vi "Dynamic Generation of Formula for Vtip.vi"(11 "Voltage (V)":T1={"Schedule"=enum."Constant", "Value"=10.0, "Start Value"=0.0, "End Value"=0.0, "Min Value"=0.0, "Max Value"=0.0, "Duty Cycle (%)"=0.0, "Signal Type"=enum."Square Wave", "Cycle Number"=0.0, "Phase (degrees)"=0.0, "formula"="1*(step(170-t)*cos(0.62831853071*t)+step(t-170)*cos(0.62831853071*(t-170))*(-1))", "formula length (nm)"=340.0, "formula resolution (nm)"=0.001}) -> (3 "Voltage (V) 2":T1={"Schedule"=enum."Constant", "Value"=10.0, "Start Value"=0.0, "End Value"=0.0, "Min Value"=0.0, "Max Value"=0.0, "Duty Cycle (%)"=0.0, "Signal Type"=enum."Square Wave", "Cycle Number"=0.0, "Phase (degrees)"=0.0, "formula"="1*(step(170-t)*cos(0.62831853071*t)+step(t-170)*cos(0.62831853071*(t-170))*(-1))", "formula length (nm)"=340.0, "formula resolution (nm)"=0.001})   [LabVIEW 2016]
uses:
  typedefs/Voltage - cluster.ctl
  typedefs/Schedule - enum.ctl
  typedefs/Signal Type - enum.ctl
  <vilib>/gmath/NI_Gmath.lvlib
panel:
  out "error":i32
  in  "formula":string="1*(step(170-t)*cos(0.62831853071*t)+step(t-170)*cos(0.62831853071*(t-170))*(-1))"
  out "XY Graph":cluster{"X Values":dbl[], "Y Values":dbl[]}(graph)
  in  "Resolution (nm)":dbl=0.001
  in  "Length (nm)":dbl=340.0
  in  "OK":bool
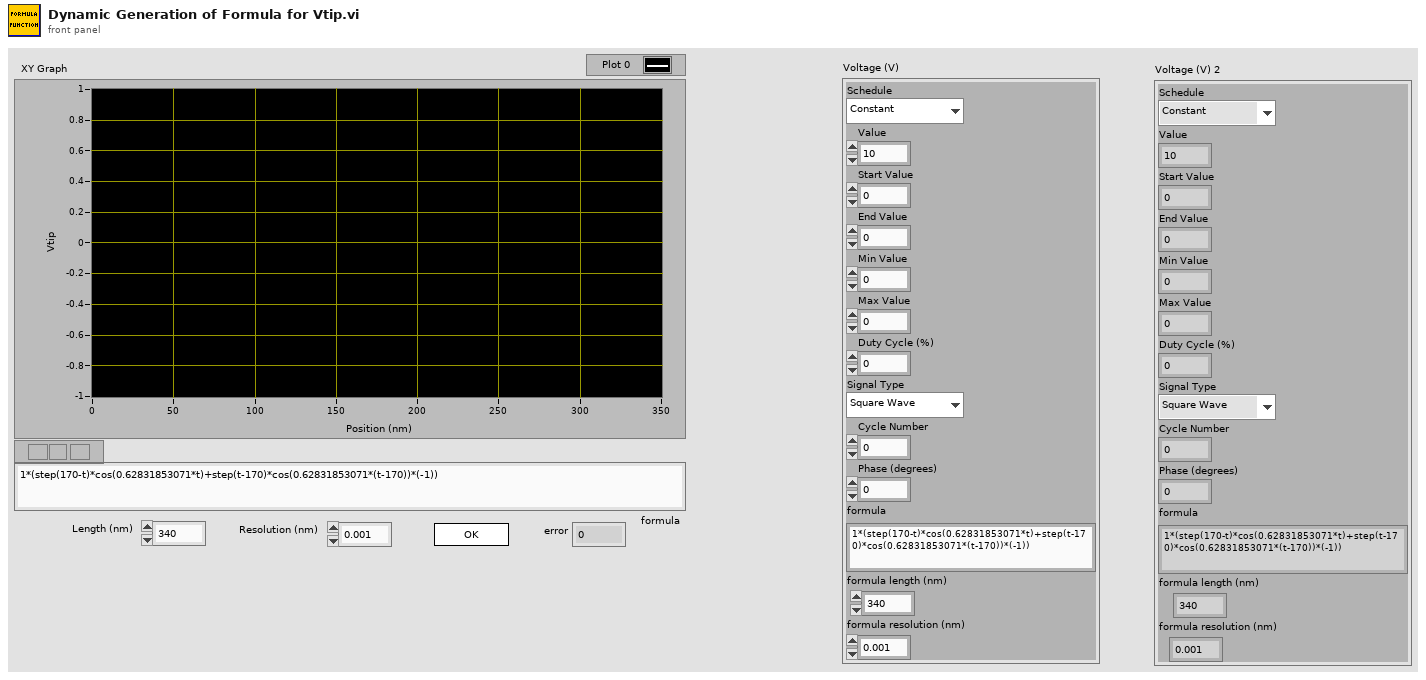
[diagram p1: front panel]
types:
  T1 = typedef "Voltage - cluster.ctl" = cluster{"Schedule":T2, "Value":dbl, "Start Value":dbl, "End Value":dbl, "Min Value":dbl, "Max Value":dbl, "Duty Cycle (%)":dbl, "Signal Type":T3, "Cycle Number":dbl, "Phase (degrees)":dbl, "formula":string, "formula length (nm)":dbl, "formula resolution (nm)":dbl}
  T2 = typedef "Schedule - enum.ctl" = enum16{"Constant", "Ramp", "Fn. Generator", "Formula"}
  T3 = typedef "Signal Type - enum.ctl" = enum16{"Sine Wave", "Triangle Wave", "Square Wave", "Sawtooth Wave"}
  T4 = enum32{"invalid app kind", "Development System", "Run Time System", "Student Edition", "Embedded LabVIEW", "Evaluation", "Custom"}
  T5 = enum32{"Invalid", "Standard", "Closed", "Hidden", "Minimized", "Maximized"}
  T6 = cluster{"Core":cluster{"Current VI Reference":refnum<vi>, "Close Panel on Exit?":bool}, "Your Boolean data":bool, "Your string data":string, "#s":u32, "Voltage (V)":T1}
  T7 = cluster{"Current VI Reference":refnum<vi>, "Close Panel on Exit?":bool}
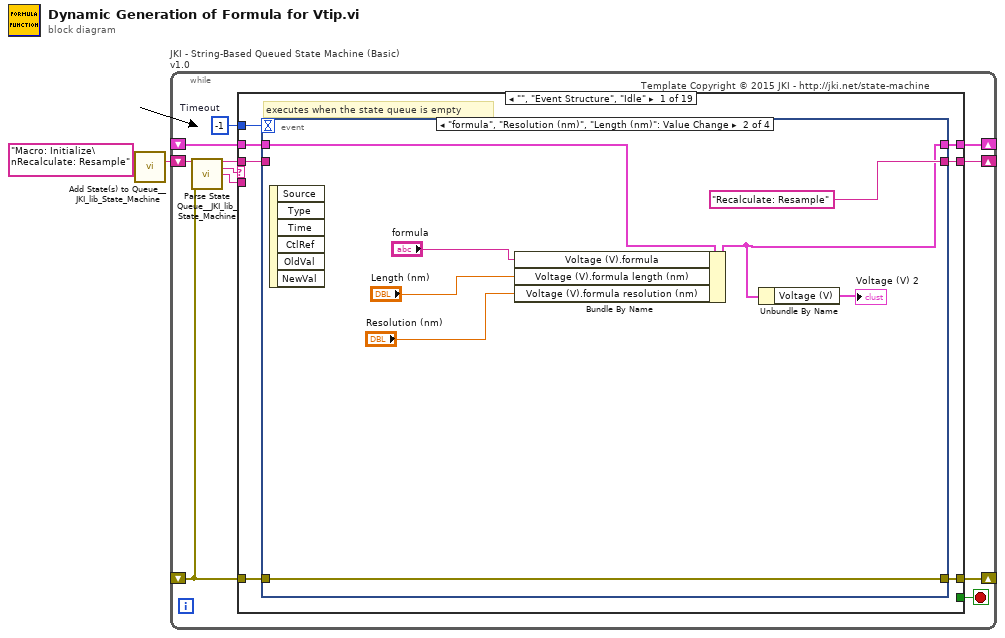
[diagram p0: block diagram]
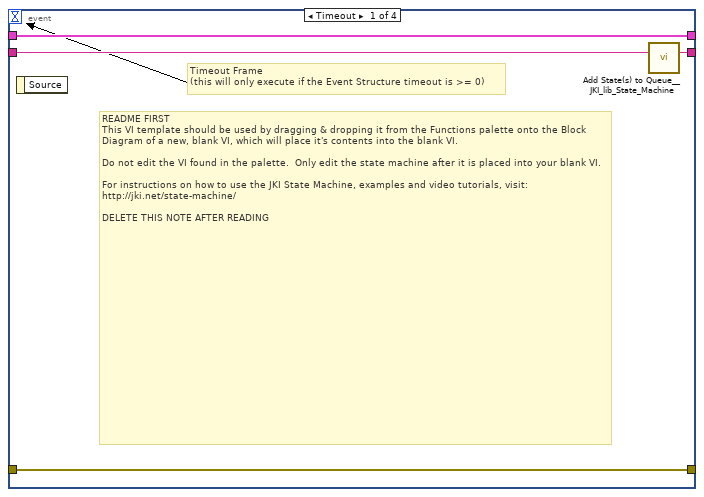
[diagram p2: hidden frame]
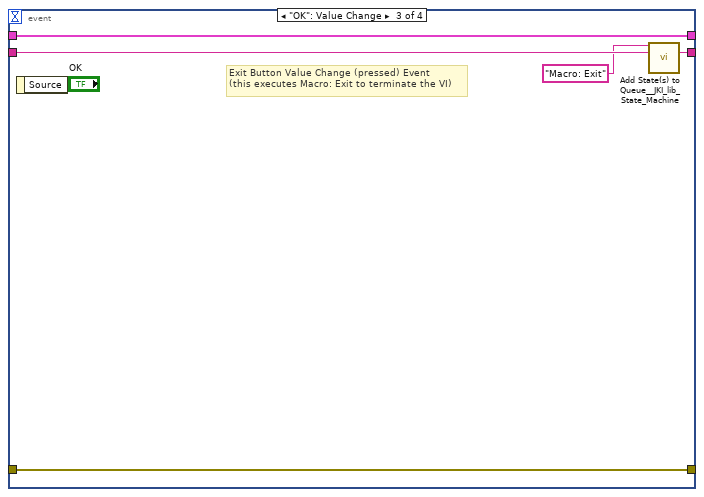
[diagram p3: hidden frame]
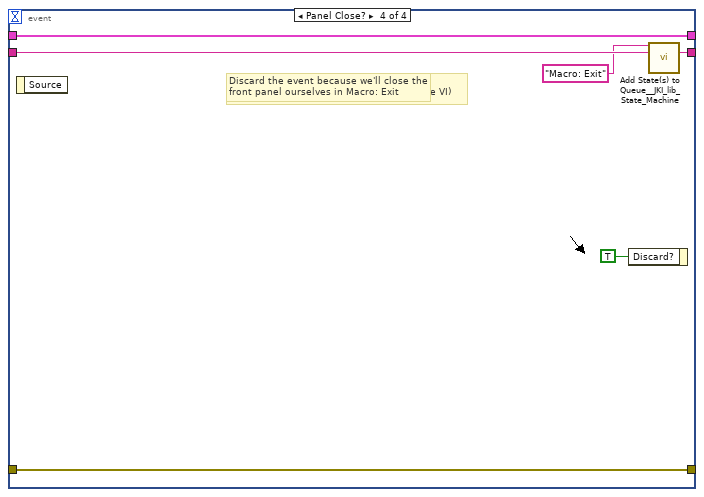
[diagram p4: hidden frame]
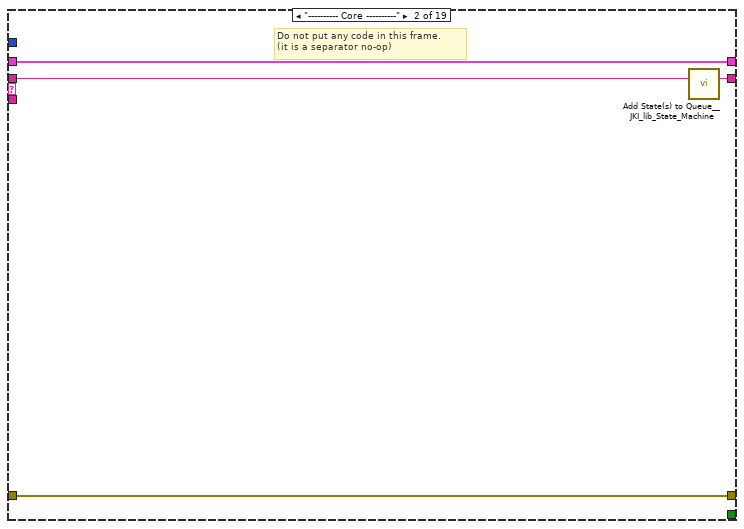
[diagram p5: hidden frame]
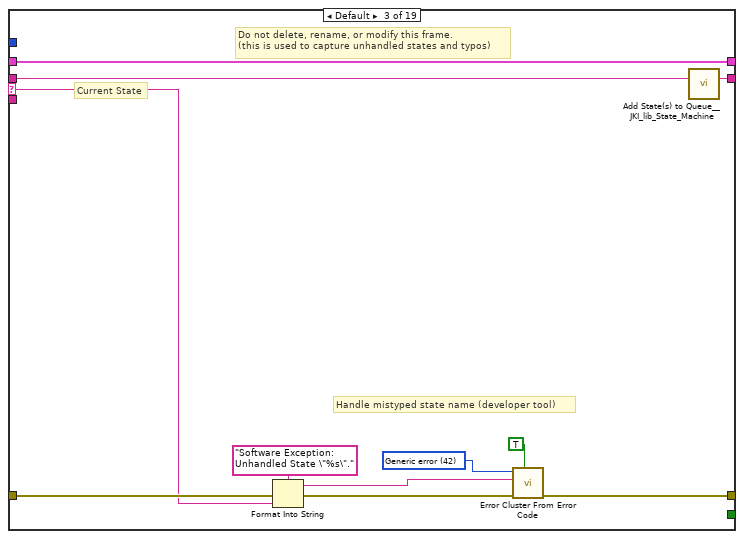
[diagram p6: hidden frame]
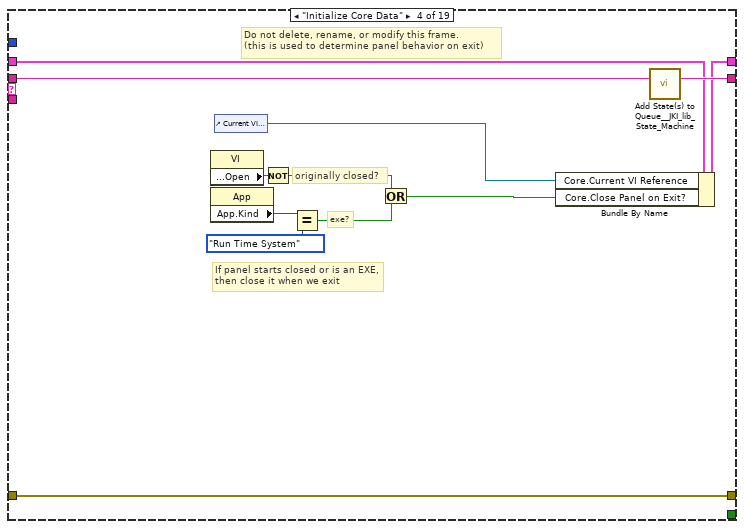
[diagram p7: hidden frame]
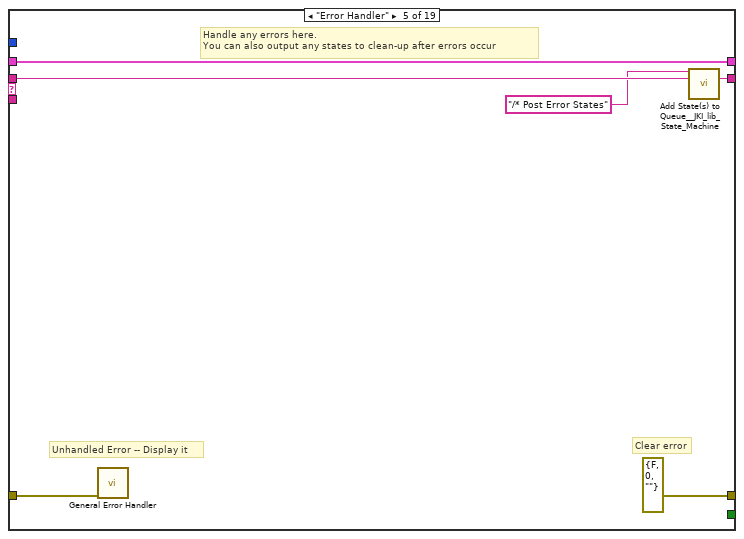
[diagram p8: hidden frame]
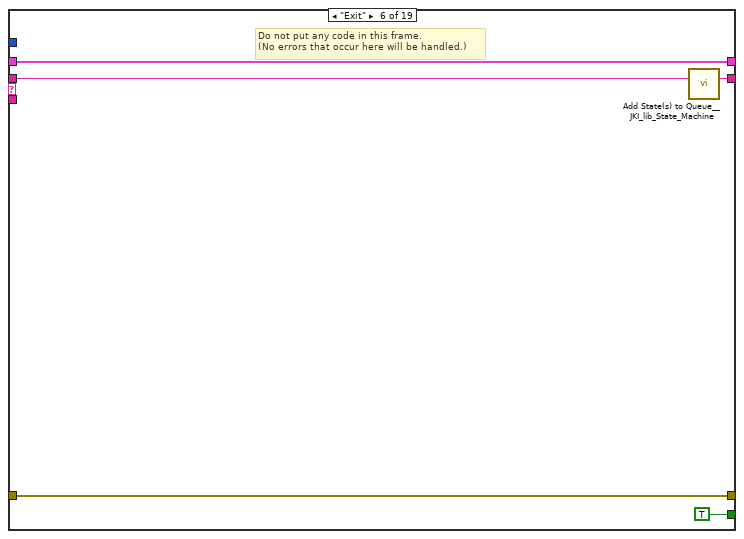
[diagram p9: hidden frame]
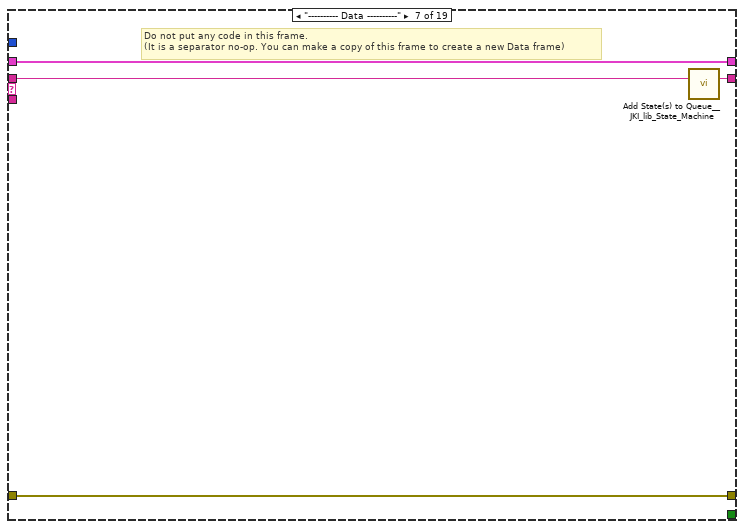
[diagram p10: hidden frame]
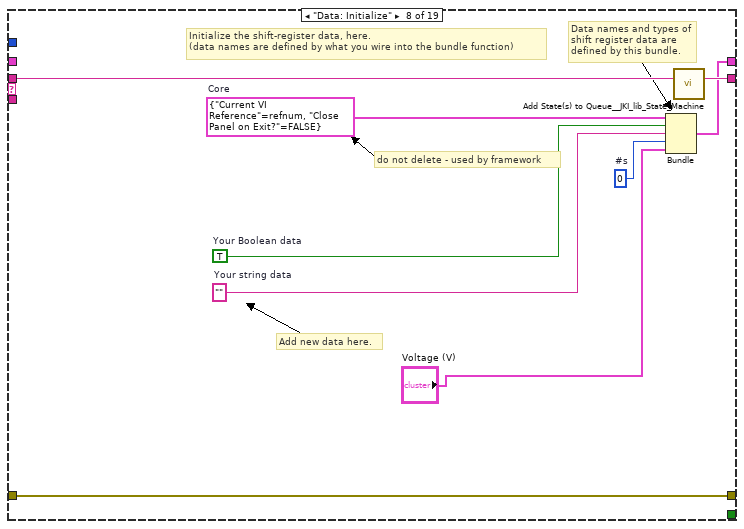
[diagram p11: hidden frame]
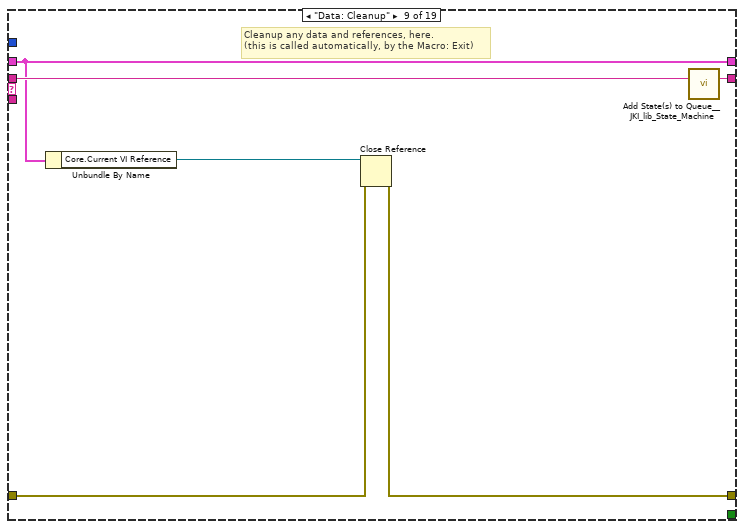
[diagram p12: hidden frame]
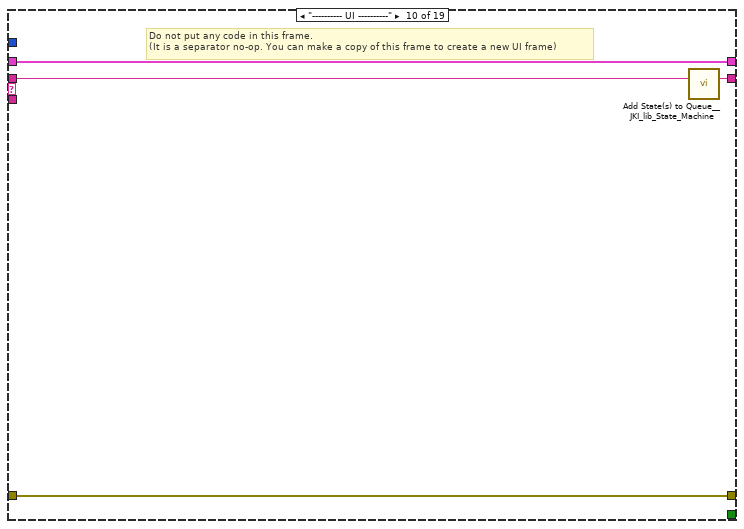
[diagram p13: hidden frame]
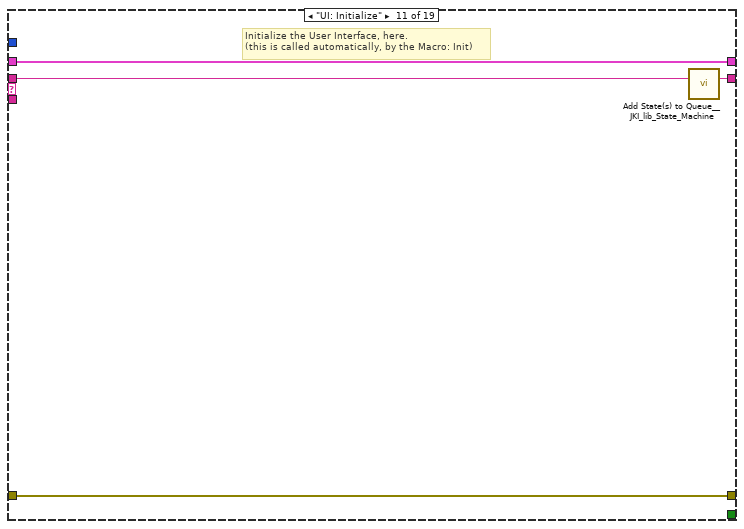
[diagram p14: hidden frame]
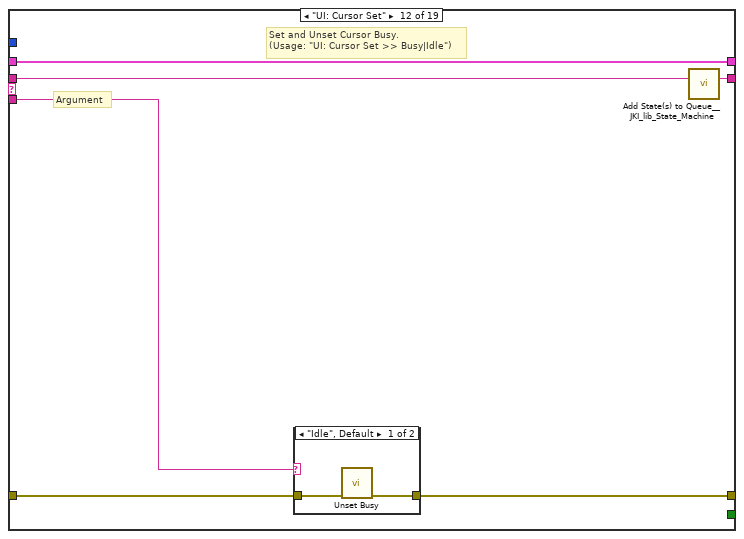
[diagram p15: hidden frame]
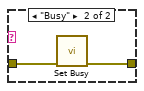
[diagram p16: hidden frame]
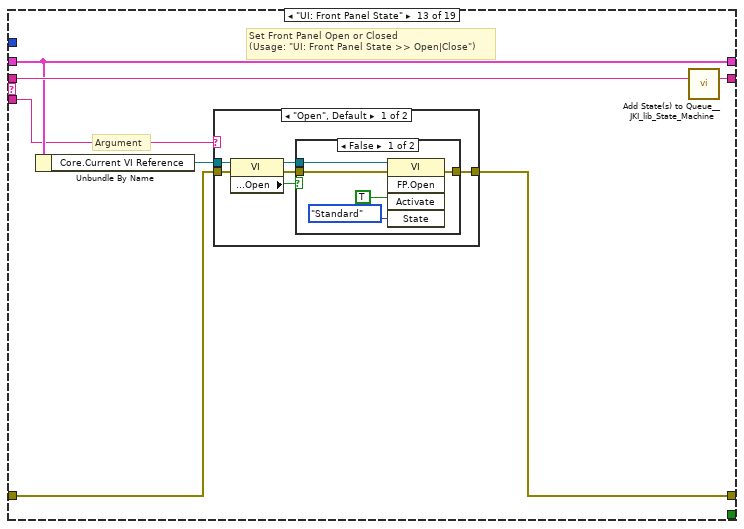
[diagram p17: hidden frame]
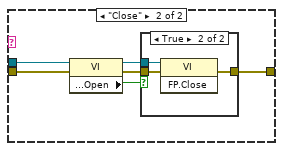
[diagram p19: hidden frame]
diagram:
  n1 = call <vilib>:"Add State(s) to Queue__JKI_lib_State_Machine.vi"("State(s) in (\"\")"="Macro: Initialize\nRecalculate: Resample") -> ("States Out"=w2:string)  [unwired: 14 in]
  n2 = while "JKI - String-Based Queued State Machine (Basic) v1.0" {
    shift-right: [w6] -> _
    shift-left: _ -> [w5]
    shift-right: [w9] -> _
    shift-left: _ -> [w3]
    shift-right: [w8] -> _
    shift-left: w2 -> [w10]
    stop <- w7 stop-if-true
    w4 = -1  # Timeout
    # "Template Copyright © 2015 JKI - http://jki.net/state-machine"
    n3 = call <vilib>:"Parse State Queue__JKI_lib_State_Machine.vi"("State Queue"=w10, "Error In (no error)"=w3) -> ("Remaining States"=w12:string, "Current State"=w13:string, "Arguments"=w11:string)  [unwired: 11 in]
    n4 = case shown="\"\", \"Event Structure\", \"Idle\"" w13 {
      selector: w13 -> [_ _ w48 _ _ _ _ _ _ _ _ _ _ _ _ _ _ _ _]
      tunnel: w12 -> [w20 w47 w52 w70 w76 w81 w85 w94 w100 w104 w108 w114 w125 w151 w156 w166 w170 w183 w187]
      tunnel: w11 -> [_ _ _ _ _ _ _ _ _ _ _ w109 w119 _ _ _ _ _ _]
      tunnel: w5 -> [w18 w44 w50 w61 w73 w79 w82 _ w95 w101 w106 w112 w121 w148 w153 w163 w167 w174 w184]
      tunnel: [w17 w45 w54 w67 errorcluster {"status"=FALSE, "code"=0, "source"=""} ("error out") w78 w83 w91 w96 w102 w105 w110 w122 w149 w154 w164 w168 w181 w185] -> w9
      tunnel: w3 -> [w16 w45 w53 w67 w72 w78 w83 w91 w97 w102 w105 w111 w123 w149 w154 w164 w168 w181 w185]
      tunnel: [w19 w46 w51 w69 w75 w80 w84 w93 w99 w103 w107 w113 w124 w150 w155 w165 w169 w182 w186] -> w8
      tunnel: [_ _ _ _ _ TRUE _ _ _ _ _ _ _ _ _ _ _ _ _] -> w7
      tunnel: [w15 w44 w50 w68 w73 w79 w82 w92 w95 w101 w106 w112 w121 w148 w153 w163 w167 w174 w184] -> w6
      tunnel: w4 -> [w14 _ _ _ _ _ _ _ _ _ _ _ _ _ _ _ _ _ _]
      frame "", "Event Structure", "Idle" {
        # "executes when the state queue is empty"
        n5 = event shown="[1] \"formula\", \"Resolution (nm)\", \"Length (nm)\": Value Change" {
          selector: _ -> [_ _ _ _]
          dyn-events: _ -> [_ _ _ _]
          timeout: w14 -> [_ _ _ _]
          tunnel: w20 -> [w24 _ w37 w43]
          tunnel: [w23 "Recalculate: Resample" w36 w42] -> w19
          tunnel: w18 -> [w21 w30 w34 w40]
          tunnel: [w22 w31 w35 w41] -> w17
          tunnel: w16 -> [w22 w31 w35 w41]
          tunnel: [w21 w26 w34 w40] -> w15
          event Timeout {
            # "README FIRST\nThis VI template should be used by dragging & dropping it from the Functions palette onto the Block Diagram of a new, blank VI, which will place it's contents into the blank VI.\n\nDo not edit the VI found in the palette.  Only edit the state machine after it is placed into your blank VI.\n\nFor instructions on how to use the JKI State Machine, examples and video tutorials, visit:\nhttp://jki.net/state-machine/\n\nDELETE THIS NOTE AFTER READING"
            # "Timeout Frame\n(this will only execute if the Event Structure timeout is >= 0)"
            n6 = event-data() -> ()  [unwired: 1 in, 1 out]
            n7 = call <vilib>:"Add State(s) to Queue__JKI_lib_State_Machine.vi"("State(s) in (\"\")"=w24) -> ("States Out"=w23:string)  [unwired: 14 in]
          }
          event "formula", "Resolution (nm)", "Length (nm)": Value Change {
            n8 = event-data() -> ()  [unwired: 1 in, 6 out]
            n9 = Bundle By Name(cluster=w30, "Voltage (V).formula"="formula", "Voltage (V).formula length (nm)"="Length (nm)", "Voltage (V).formula resolution (nm)"="Resolution (nm)") -> (w26:T6)
            n10 = Unbundle By Name(w26) -> ("Voltage (V)"=→"Voltage (V) 2":T1)
          }
          event "OK": Value Change {
            # "Exit Button Value Change (pressed) Event\n(this executes Macro: Exit to terminate the VI)"
            n11 = event-data() -> ()  [unwired: 1 in, 1 out]
            n12 = call <vilib>:"Add State(s) to Queue__JKI_lib_State_Machine.vi"("State(s) in Front (\"\")"="Macro: Exit", "State(s) in (\"\")"=w37) -> ("States Out"=w36:string)  [unwired: 13 in]
          }
          event Panel Close? {
            # "Discard the event because we'll close the front panel ourselves in Macro: Exit"
            # "Close Panel button (pressed) Event\n(this executes Macro: Exit to terminate the VI)"
            n13 = event-data() -> ()  [unwired: 1 in, 1 out]
            n14 = event-data("Discard?"=TRUE) -> ()  [unwired: 1 in, 1 out]
            n15 = call <vilib>:"Add State(s) to Queue__JKI_lib_State_Machine.vi"("State(s) in Front (\"\")"="Macro: Exit", "State(s) in (\"\")"=w43) -> ("States Out"=w42:string)  [unwired: 13 in]
          }
        }
      }
      frame "---------- Core ----------" {
        # "Do not put any code in this frame.\n(it is a separator no-op)"
        n16 = call <vilib>:"Add State(s) to Queue__JKI_lib_State_Machine.vi"("State(s) in (\"\")"=w47) -> ("States Out"=w46:string)  [unwired: 14 in]
      }
      frame Default {
        w57 = 42 items=["No error", "Argument error", "Memory is full", "Out of zone", "End of file", "File already open", "Generic file I/O error", "File not found", "File permission error", "Disk is full", "Duplicate path", "Too many files open", "System feature not enabled", "Resource file not found", "Cannot add resource", "Resource not found", "Image not found", "Image memory error", "Pen does not exist", "Config type invalid", "Config token not found", "Config parse error", "Config memory error", "Bad external code format", "Bad external code offset", "External code not present", "Null window", "Destroy window error", "Null menu", "Print aborted", "Bad print record", "Print driver error", "Windows error during printing", "Memory error during printing", "Print dialog error", "Generic print error", "Invalid device refnum", "Device not found", "Device parameter error", "Device unit error", "Cannot open device", "Device call aborted", "Generic error", "Cancelled by user", "Object ID too low", "Object ID too high", "Object not in heap", "Unknown heap", "Unknown object (invalid DefProc)", "Unknown object (DefProc not in table)", "Message out of range", "Invalid (null) method", "Unknown message", "Manager call not supported", "Bad address", "Network operation in progress", "Network operation timed out", "Connection is busy", "Network attribute not supported", "Network error", "Address in use", "System out of memory", "Connection aborted", "Connection refused", "Not connected", "Already connected", "Connection closed", "Initialization error (interapplication manager)", "Bad occurrence", "Wait on unbound occurrence handler", "Occurrence queue overflow", "Datalog type conflict", "Unused", "Unrecognized type (interapplication manager)", "Memory corrupt", "Failed to make temporary DLL", "Old CIN version", "Drag socket not found", "Failed to load drop-object", "Failed to register OLE object", "Failed to release OLE object", "Format specifier type mismatch", "Unknown format specifier", "Too few format specifiers", "Too many format specifiers", "Scan failed", "Newer CIN version", "Error converting to variant", "Runtime menu error", "Password tampered", "Variant attribute not found", "Incompatible variant data type", "Event data is not available", "Event Store is not present", "Occurrence is not found", "Event Queue is not created", "Event info is not available", "Refnum passed is NULL", "Error retrieving Class GUID", "Error retrieving CoClass GUID", "Error retrieving TypeLib GUID.", "Bad built application magic bytes.", "Specific driver is different from the specific driver associated with the Logical Name.", "There is no session opened to the class driver.", "Max Error", "MAX - Error with config objects", "MAX - Error loading configuration", "MAX - Group not supported"]
        # "Current State"
        # "Do not delete, rename, or modify this frame.\n(this is used to capture unhandled states and typos)"
        # "Handle mistyped state name (developer tool)"
        n17 = Format Into String(format string="Software Exception: Unhandled State \"%s\"." ("message"), error in=w53, w48) -> (resulting string=w56:string, error out=w55:errorcluster)  [unwired: 1 in]
        n18 = call <vilib>:"Error Cluster From Error Code.vi"("show call chain? (False)"=TRUE, "error in (no error)"=w55, "error message (\"\")"=w56, "error code (0)"=w57) -> ("error out"=w54:errorcluster)  [unwired: 5 in]
        n19 = call <vilib>:"Add State(s) to Queue__JKI_lib_State_Machine.vi"("State(s) in (\"\")"=w52) -> ("States Out"=w51:string)  [unwired: 14 in]
      }
      frame "Initialize Core Data" {
        # "Do not delete, rename, or modify this frame.\n(this is used to determine panel behavior on exit)"
        # "originally closed?"
        # "exe?"
        # "If panel starts closed or is an EXE, then close it when we exit"
        n20 = property class="VI"() -> ("Front Panel.Open"=w66:bool)  [unwired: 2 in, 2 out]
        n21 = property class="App"() -> ("App.Kind"=w65:T4)  [unwired: 2 in, 2 out]
        n22 = control-ref of="Current VI Reference"() -> (w59:refnum<vi>)
        n23 = Not(x=w66) -> (.not. x?=w63:bool)
        n24 = Equal?(x=w65, y=T4."Run Time System" ("Application:Kind")) -> (x = y?=w62:bool)
        n25 = Or(x=w63, y=w62) -> (x .or. y?=w60:bool)
        n26 = Bundle By Name(cluster=w61, "Core.Current VI Reference"=w59, "Core.Close Panel on Exit?"=w60) -> (w68:T6)
        n27 = call <vilib>:"Add State(s) to Queue__JKI_lib_State_Machine.vi"("State(s) in (\"\")"=w70) -> ("States Out"=w69:string)  [unwired: 14 in]
      }
      frame "Error Handler" {
        # "Unhandled Error -- Display it"
        # "Handle any errors here.\nYou can also output any states to clean-up after errors occur"
        # "Clear error"
        n28 = call <vilib>:"General Error Handler.vi"("error in (no error)"=w72) -> ()  [unwired: 10 in, 5 out]
        n29 = call <vilib>:"Add State(s) to Queue__JKI_lib_State_Machine.vi"("State(s) in Front (\"\")"="/* Post Error States", "State(s) in (\"\")"=w76) -> ("States Out"=w75:string)  [unwired: 13 in]
      }
      frame "Exit" {
        # "Do not put any code in this frame.\n(No errors that occur here will be handled.)"
        n30 = call <vilib>:"Add State(s) to Queue__JKI_lib_State_Machine.vi"("State(s) in (\"\")"=w81) -> ("States Out"=w80:string)  [unwired: 14 in]
      }
      frame "---------- Data ----------" {
        # "Do not put any code in this frame.\n(It is a separator no-op. You can make a copy of this frame to create a new Data frame)"
        n31 = call <vilib>:"Add State(s) to Queue__JKI_lib_State_Machine.vi"("State(s) in (\"\")"=w85) -> ("States Out"=w84:string)  [unwired: 14 in]
      }
      frame "Data: Initialize" {
        w87 = u32 0  # #s
        w88 = T7 {"Current VI Reference"=refnum, "Close Panel on Exit?"=FALSE}  # Core
        w90 = TRUE  # Your Boolean data
        w89 = ""  # Your string data
        # "do not delete - used by framework"
        # "Add new data here."
        # "Data names and types of shift register data are defined by this bundle."
        # "Initialize the shift-register data, here.\n(data names are defined by what you wire into the bundle function)"
        n32 = Bundle("Core"=w88, "Your Boolean data"=w90, "Your string data"=w89, "#s"=w87, "Voltage (V)"="Voltage (V)") -> (w92:T6)  [unwired: 1 in]
        n33 = call <vilib>:"Add State(s) to Queue__JKI_lib_State_Machine.vi"("State(s) in (\"\")"=w94) -> ("States Out"=w93:string)  [unwired: 14 in]
      }
      frame "Data: Cleanup" {
        # "Cleanup any data and references, here.\n(this is called automatically, by the Macro: Exit)"
        n34 = Unbundle By Name(w95) -> ("Core.Current VI Reference"=w98:refnum<vi>)
        n35 = Close Reference(reference=w98, error in (no error)=w97) -> (error out=w96:errorcluster)
        n36 = call <vilib>:"Add State(s) to Queue__JKI_lib_State_Machine.vi"("State(s) in (\"\")"=w100) -> ("States Out"=w99:string)  [unwired: 14 in]
      }
      frame "---------- UI ----------" {
        # "Do not put any code in this frame.\n(It is a separator no-op. You can make a copy of this frame to create a new UI frame)"
        n37 = call <vilib>:"Add State(s) to Queue__JKI_lib_State_Machine.vi"("State(s) in (\"\")"=w104) -> ("States Out"=w103:string)  [unwired: 14 in]
      }
      frame "UI: Initialize" {
        # "Initialize the User Interface, here.\n(this is called automatically, by the Macro: Init)"
        n38 = call <vilib>:"Add State(s) to Queue__JKI_lib_State_Machine.vi"("State(s) in (\"\")"=w108) -> ("States Out"=w107:string)  [unwired: 14 in]
      }
      frame "UI: Cursor Set" {
        # "Argument"
        # "Set and Unset Cursor Busy.\n(Usage: \"UI: Cursor Set >> Busy|Idle\")"
        n39 = case shown="\"Idle\", Default" w109 {
          tunnel: w111 -> [w116 w118]
          tunnel: [w115 w117] -> w110
          frame "Idle", Default {
            n40 = call <vilib>:"Unset Busy.vi"("error in (no error)"=w116) -> ("error out"=w115:errorcluster)  [unwired: 10 in]
          }
          frame "Busy" {
            n41 = call <vilib>:"Set Busy.vi"("error in (no error)"=w118) -> ("error out"=w117:errorcluster)  [unwired: 9 in, 1 out]
          }
        }
        n42 = call <vilib>:"Add State(s) to Queue__JKI_lib_State_Machine.vi"("State(s) in (\"\")"=w114) -> ("States Out"=w113:string)  [unwired: 14 in]
      }
      frame "UI: Front Panel State" {
        # "Argument"
        # "Set Front Panel Open or Closed\n(Usage: \"UI: Front Panel State >> Open|Close\")"
        n43 = Unbundle By Name(w121) -> ("Core.Current VI Reference"=w120:refnum<vi>)
        n44 = case shown="\"Open\", Default" w119 {
          tunnel: w123 -> [w129 w142]
          tunnel: [w131 w143] -> w122
          tunnel: w120 -> [w130 w140]
          frame "Open", Default {
            n45 = property class="VI"(reference=w130, error in=w129) -> (reference out=w127:refnum<vi>, error out=w128:errorcluster, "Front Panel.Open"=w126:bool)
            n46 = case shown="False" w126 {
              tunnel: [w134 w137] -> w131
              tunnel: w128 -> [w133 w137]
              tunnel: w127 -> [w132 _]
              frame False {
                n47 = invoke class="VI" method="FP.Open"(reference=w132, error in=w133, "Activate"=TRUE, "State"=T5."Standard") -> (error out=w134:errorcluster)  [unwired: 1 in, 4 out]
              }
              frame True {
              }
            }
          }
          frame "Close" {
            n48 = property class="VI"(reference=w140, error in=w142) -> (reference out=w139:refnum<vi>, error out=w141:errorcluster, "Front Panel.Open"=w138:bool)
            n49 = case shown="True" w138 {
              tunnel: [w144 w147] -> w143
              tunnel: w141 -> [w144 w146]
              tunnel: w139 -> [_ w145]
              frame False {
              }
              frame True {
                n50 = invoke class="VI" method="FP.Close"(reference=w145, error in=w146) -> (error out=w147:errorcluster)  [unwired: 1 in, 2 out]
              }
            }
          }
        }
        n51 = call <vilib>:"Add State(s) to Queue__JKI_lib_State_Machine.vi"("State(s) in (\"\")"=w125) -> ("States Out"=w124:string)  [unwired: 14 in]
      }
      frame "---------- Macro ----------" {
        # "Do not put any code in this frame.\n(It is a separator no-op. You can make a copy of this frame to create a new Macro frame)"
        n52 = call <vilib>:"Add State(s) to Queue__JKI_lib_State_Machine.vi"("State(s) in (\"\")"=w151) -> ("States Out"=w150:string)  [unwired: 14 in]
      }
      frame "Macro: Initialize" {
        w152 = "Data: Initialize\nInitialize Core Data\nUI: Initialize\nUI: Front Panel State >> Open"  # Data: Initialize Initialize Core Data UI: Initialize UI: Front Panel State >> Open
        # "Initialization Macro\n(This is called once, when the VI starts)"
        n53 = call <vilib>:"Add State(s) to Queue__JKI_lib_State_Machine.vi"("State(s) in Front (\"\")"=w152, "State(s) in (\"\")"=w156) -> ("States Out"=w155:string)  [unwired: 13 in]
      }
      frame "Macro: Exit" {
        # "Exit Macro\n(This is called once, when the VI exits)"
        n54 = Unbundle By Name(w163) -> ("Core.Close Panel on Exit?"=w162:bool)
        n55 = Select(t="UI: Front Panel State >> Close", s=w162, f="") -> (s? t:f=w159:string)
        n56 = call <vilib>:"Add State(s) to Queue__JKI_lib_State_Machine.vi"("State(s) in (\"\")"=w159, "State(s) at Back (\"\")"="Data: Cleanup\nExit") -> ("States Out"=w157:string)  [unwired: 13 in]
        n57 = call <vilib>:"Add State(s) to Queue__JKI_lib_State_Machine.vi"("State(s) in Front (\"\")"=w157, "State(s) in (\"\")"=w166) -> ("States Out"=w165:string)  [unwired: 13 in]
      }
      frame "---------- Recalculate ----------" {
        # "Template Separator\n(You can make a copy of, or modify, this frame)"
        n58 = call <vilib>:"Add State(s) to Queue__JKI_lib_State_Machine.vi"("State(s) in (\"\")"=w170) -> ("States Out"=w169:string)  [unwired: 14 in]
      }
      frame "Recalculate: Resample" {
        # "Your code here.\n(You can make a copy of, or modify, this frame)"
        n59 = Unbundle By Name(w174) -> ("Voltage (V).formula"=w173:string, "Voltage (V).formula length (nm)"=w171:dbl, "Voltage (V).formula resolution (nm)"=w172:dbl)
        n60 = Divide(x=w171, y=w172) -> (x/y=w176:dbl)
        n61 = call <vilib>:"Eval y=f(x).vi"("formula"=w173, "end"=w171, "start"=0.0, "number of points"=w176) -> ("error"=→"error":i32, "Y Values"=w179:dbl[], "X Values"=w180:dbl[])  [unwired: 1 out]
        n62 = Bundle("X Values"=w180, "Y Values"=w179) -> (→"XY Graph":cluster{"X Values":dbl[], "Y Values":dbl[]})  [unwired: 1 in]
        n63 = call <vilib>:"Add State(s) to Queue__JKI_lib_State_Machine.vi"("State(s) in (\"\")"=w183) -> ("States Out"=w182:string)  [unwired: 14 in]
      }
      frame "New Category: 2" {
        # "Your code here.\n(You can make a copy of, or modify, this frame)"
        n64 = call <vilib>:"Add State(s) to Queue__JKI_lib_State_Machine.vi"("State(s) in (\"\")"=w187) -> ("States Out"=w186:string)  [unwired: 14 in]
      }
    }
  }
